vi "Assist Sampling Setup Panel.vi"(8 "error in":errorcluster, 10 "fs in [Hz]":dbl, 11 "session in":T2={"adc"={"niScope"={"channel cfg"=[], "sessions"=[], "multi cards"=FALSE, "channels"=0, "type"=enum."n/a", "memory [B/chn]"=0, "ext. clock [Hz]"=0.0, "samples count"=0, "use streaming"=FALSE, "proc setup"={"packet size [smpl]"=0, "current timeout [s]"=0.0, "blk2blk timeout [s]"=0.0, "event time"=timestamp(0 s since 1904-01-01), "temp sampl T [s]"=0.0, "data queue"=refnum, "stop notifier"=refnum, "proc ref"=refnum}, "sample width [B]"=0, "ranges [V]"=[], "trigger setup"={"coupling"=1, "level [V]"=0.0, "slope"=0, "mode"=enum."Immediate"}, "fs [Hz]"=0.0, "bitres [bit]"=0}, "3458A"={"channels"=[], "sync unit"={"VISA"="", "type"=enum."Picotest U6200A"}, "awg unit"={"type"=enum."Agilent 331xxA to 332xxA", "VISA"="", "enable 10MHz ref"=FALSE}, "sync mode"=enum."MASTER-SLAVE, MASTER clocked by TIMER", "streaming mode"=FALSE, "idn mode"=enum."Auto", "sampling mode"=enum."DCV", "Ts [s]"=0.0, "sample memory [B]"=0, "proc setup"={"channel id"=0, "packet size [smpl]"=0, "current timeout [s]"=0.0, "blk2blk timeout [s]"=0.0, "event time"=timestamp(0 s since 1904-01-01), "stop notifier"=refnum, "data queues"=[], "proc refs"=[], "bus semaphore"=refnum}, "sample size [B]"=0, "sample count"=0, "aux data"={"channel id"=0, "valid?"=[], "gain [V]"=[], "timestamp [s]"=[], "Ts [s]"=0.0, "abs timestamp"=timestamp(0 s since 1904-01-01), "t [deg C]"=[]}, "ranges [V]"=[], "aperture [s]"=0.0, "LEVEL trigger"={"edge"=enum."POS", "level [V]"=0.0, "coupling"=enum."DC"}, "trigger mode"=enum."AUTO", "measure temp.?"=FALSE, "disp mesages"=[], "shared bus?"=FALSE, "disable display?"=FALSE, "aper mode"=enum."Manual", "aper rules"=[]}, "dsdll"={"dsdll"={"dsdll path"=path "", "dsdll handle"=[], "output devices"=[], "capture devices"=[]}, "channels"=0, "device id"=0, "channel idns"=[], "proc setup"={"packet size [smpl]"=0, "current timeout [s]"=0.0, "blk2blk timeout [s]"=0.0, "event time"=timestamp(0 s since 1904-01-01), "data queue"=refnum, "stop notifier"=refnum, "proc ref"=refnum}, "samples count"=0, "fs [Hz]"=0.0}, "type"=enum."niScope", "channel idn str"=[], "aux instr idn str"=[], "modified?"=FALSE, "simadc"={"channels"=[], "range [V]"=0.0, "Ts step [s]"=0.0, "time [s]"=0.0, "fs [Hz]"=0.0, "count"=0, "smpl offset"=0, "set count"=0, "bit res"=0}, "force rst?"=FALSE, "exit mode"=enum."Immediate reset", "exit dly"=0.0, "exit tmr"=timestamp(0 s since 1904-01-01), "busy?"=FALSE, "accessed?"=FALSE, "QuADC session"={"channel cfg"=[], "sessions"=[], "multi cards"=FALSE, "channels"=0, "type"=enum."n/a", "memory [B/chn]"=0, "ext. clock [Hz]"=0.0, "samples count"=0, "use streaming"=FALSE, "proc setup"={"packet size [smpl]"=0, "current timeout [s]"=0.0, "blk2blk timeout [s]"=0.0, "event time"=timestamp(0 s since 1904-01-01), "temp sampl T [s]"=0.0, "data queue"=refnum, "stop notifier"=refnum, "proc ref"=refnum}, "sample width [B]"=0, "ranges [V]"=[], "trigger setup"={"coupling"=1, "level [V]"=0.0, "slope"=0, "mode"=enum."Immediate"}, "fs [Hz]"=0.0, "bitres [bit]"=0}}, "sequence"=[], "sequence setup"={"group setups"=[], "average cycles"=0, "range mode"=enum."Keep defaults", "fs mode"=enum."Frequency", "rng even"=0.0, "rng odd"=0.0, "folder"=path "", "name base"="", "meas id"=0, "settle [s]"=0.0}, "golpi"=refnum, "processing setup"={"mode"=enum."Raw", "call after avgs?"=FALSE, "calculate?"=FALSE, "raw mode"={"command"="", "result mode"=enum."Display console output (only Octave)", "res variable"=""}, "QWTB"={"QWTB path"=path "", "alg filter path"="", "alg ids"=[], "alg parameters"=[], "parsed parameters"=[], "selected alg id"="", "selected unc mode"=enum."None", "qwtb mcc"=100, "qwtb timeout"=90, "qwtb covg"=95.0, "qwtb ofs"=0, "qwtb lim data"=0, "multicore"={"jobs folder"=path "", "cores"=0, "max jobs"=0, "mode"=enum."Singlecore"}, "unc once?"=FALSE}}, "corrections"={"transducers"={"channels"=[], "last path"=path ""}, "digitizer"={"last path"=path "", "channel paths"=[], "channel idns"=[], "correction name"="", "channel names"=[], "folders to copy"=[], "channel valid"=[], "correction path"=path "", "correction rel path"="", "rel folders to copy"=[]}}, "assist cfg"={"P"=0, "Q"=0, "rel shift"=0.0, "ref freq"=0.0, "min fs"=0.0, "max fs tol"=0.0, "min int"=0.0, "max int"=0.0, "max err"=0.0, "max timeout"=0.0}} {"corrections"."transducers"."channels"."Phase index" min=1 step=1; "adc"."QuADC session"."trigger setup"."level [V]" format="%.2f"; "adc"."QuADC session"."trigger setup"."coupling" items=["AC"=0, "DC"=1, "HF Reject"=3, "LF Reject"=4, "AC Plus HF Reject"=1001]; "adc"."QuADC session"."channel cfg"."Clock fr. (Hz)" min=0.0 format="%#_9p"; "adc"."QuADC session"."channel cfg"."Number of JJ" min=1; "adc"."QuADC session"."channel cfg"."Range [Vpk]" min=0.0; "adc"."QuADC session"."channel cfg"."Channel" min=0; "adc"."3458A"."channels"."Range [Vpk]" min=0.0; "adc"."niScope"."trigger setup"."level [V]" format="%.2f"; "adc"."niScope"."trigger setup"."coupling" items=["AC"=0, "DC"=1, "HF Reject"=3, "LF Reject"=4, "AC Plus HF Reject"=1001]; "adc"."niScope"."channel cfg"."Range [Vpk]" min=0.0; "adc"."niScope"."channel cfg"."Channel" min=0}) -> (0 "error out":errorcluster, 1 "ok":bool, 2 "smpl setup":T1, 3 "session out":T2={"adc"={"niScope"={"channel cfg"=[], "sessions"=[], "multi cards"=FALSE, "channels"=0, "type"=enum."n/a", "memory [B/chn]"=0, "ext. clock [Hz]"=0.0, "samples count"=0, "use streaming"=FALSE, "proc setup"={"packet size [smpl]"=0, "current timeout [s]"=0.0, "blk2blk timeout [s]"=0.0, "event time"=timestamp(0 s since 1904-01-01), "temp sampl T [s]"=0.0, "data queue"=refnum, "stop notifier"=refnum, "proc ref"=refnum}, "sample width [B]"=0, "ranges [V]"=[], "trigger setup"={"coupling"=1, "level [V]"=0.0, "slope"=0, "mode"=enum."Immediate"}, "fs [Hz]"=0.0, "bitres [bit]"=0}, "3458A"={"channels"=[], "sync unit"={"VISA"="", "type"=enum."Picotest U6200A"}, "awg unit"={"type"=enum."Agilent 331xxA to 332xxA", "VISA"="", "enable 10MHz ref"=FALSE}, "sync mode"=enum."MASTER-SLAVE, MASTER clocked by TIMER", "streaming mode"=FALSE, "idn mode"=enum."Auto", "sampling mode"=enum."DCV", "Ts [s]"=0.0, "sample memory [B]"=0, "proc setup"={"channel id"=0, "packet size [smpl]"=0, "current timeout [s]"=0.0, "blk2blk timeout [s]"=0.0, "event time"=timestamp(0 s since 1904-01-01), "stop notifier"=refnum, "data queues"=[], "proc refs"=[], "bus semaphore"=refnum}, "sample size [B]"=0, "sample count"=0, "aux data"={"channel id"=0, "valid?"=[], "gain [V]"=[], "timestamp [s]"=[], "Ts [s]"=0.0, "abs timestamp"=timestamp(0 s since 1904-01-01), "t [deg C]"=[]}, "ranges [V]"=[], "aperture [s]"=0.0, "LEVEL trigger"={"edge"=enum."POS", "level [V]"=0.0, "coupling"=enum."DC"}, "trigger mode"=enum."AUTO", "measure temp.?"=FALSE, "disp mesages"=[], "shared bus?"=FALSE, "disable display?"=FALSE, "aper mode"=enum."Manual", "aper rules"=[]}, "dsdll"={"dsdll"={"dsdll path"=path "", "dsdll handle"=[], "output devices"=[], "capture devices"=[]}, "channels"=0, "device id"=0, "channel idns"=[], "proc setup"={"packet size [smpl]"=0, "current timeout [s]"=0.0, "blk2blk timeout [s]"=0.0, "event time"=timestamp(0 s since 1904-01-01), "data queue"=refnum, "stop notifier"=refnum, "proc ref"=refnum}, "samples count"=0, "fs [Hz]"=0.0}, "type"=enum."niScope", "channel idn str"=[], "aux instr idn str"=[], "modified?"=FALSE, "simadc"={"channels"=[], "range [V]"=0.0, "Ts step [s]"=0.0, "time [s]"=0.0, "fs [Hz]"=0.0, "count"=0, "smpl offset"=0, "set count"=0, "bit res"=0}, "force rst?"=FALSE, "exit mode"=enum."Immediate reset", "exit dly"=0.0, "exit tmr"=timestamp(0 s since 1904-01-01), "busy?"=FALSE, "accessed?"=FALSE, "QuADC session"={"channel cfg"=[], "sessions"=[], "multi cards"=FALSE, "channels"=0, "type"=enum."n/a", "memory [B/chn]"=0, "ext. clock [Hz]"=0.0, "samples count"=0, "use streaming"=FALSE, "proc setup"={"packet size [smpl]"=0, "current timeout [s]"=0.0, "blk2blk timeout [s]"=0.0, "event time"=timestamp(0 s since 1904-01-01), "temp sampl T [s]"=0.0, "data queue"=refnum, "stop notifier"=refnum, "proc ref"=refnum}, "sample width [B]"=0, "ranges [V]"=[], "trigger setup"={"coupling"=1, "level [V]"=0.0, "slope"=0, "mode"=enum."Immediate"}, "fs [Hz]"=0.0, "bitres [bit]"=0}}, "sequence"=[], "sequence setup"={"group setups"=[], "average cycles"=0, "range mode"=enum."Keep defaults", "fs mode"=enum."Frequency", "rng even"=0.0, "rng odd"=0.0, "folder"=path "", "name base"="", "meas id"=0, "settle [s]"=0.0}, "golpi"=refnum, "processing setup"={"mode"=enum."Raw", "call after avgs?"=FALSE, "calculate?"=FALSE, "raw mode"={"command"="", "result mode"=enum."Display console output (only Octave)", "res variable"=""}, "QWTB"={"QWTB path"=path "", "alg filter path"="", "alg ids"=[], "alg parameters"=[], "parsed parameters"=[], "selected alg id"="", "selected unc mode"=enum."None", "qwtb mcc"=100, "qwtb timeout"=90, "qwtb covg"=95.0, "qwtb ofs"=0, "qwtb lim data"=0, "multicore"={"jobs folder"=path "", "cores"=0, "max jobs"=0, "mode"=enum."Singlecore"}, "unc once?"=FALSE}}, "corrections"={"transducers"={"channels"=[], "last path"=path ""}, "digitizer"={"last path"=path "", "channel paths"=[], "channel idns"=[], "correction name"="", "channel names"=[], "folders to copy"=[], "channel valid"=[], "correction path"=path "", "correction rel path"="", "rel folders to copy"=[]}}, "assist cfg"={"P"=0, "Q"=0, "rel shift"=0.0, "ref freq"=0.0, "min fs"=0.0, "max fs tol"=0.0, "min int"=0.0, "max int"=0.0, "max err"=0.0, "max timeout"=0.0}} {"corrections"."transducers"."channels"."Phase index" min=1 step=1; "adc"."QuADC session"."trigger setup"."level [V]" format="%.2f"; "adc"."QuADC session"."trigger setup"."coupling" items=["AC"=0, "DC"=1, "HF Reject"=3, "LF Reject"=4, "AC Plus HF Reject"=1001]; "adc"."QuADC session"."channel cfg"."Clock fr. (Hz)" min=0.0 format="%#_9p"; "adc"."QuADC session"."channel cfg"."Number of JJ" min=1; "adc"."QuADC session"."channel cfg"."Range [Vpk]" min=0.0; "adc"."QuADC session"."channel cfg"."Channel" min=0; "adc"."3458A"."channels"."Range [Vpk]" min=0.0; "adc"."niScope"."trigger setup"."level [V]" format="%.2f"; "adc"."niScope"."trigger setup"."coupling" items=["AC"=0, "DC"=1, "HF Reject"=3, "LF Reject"=4, "AC Plus HF Reject"=1001]; "adc"."niScope"."channel cfg"."Range [Vpk]" min=0.0; "adc"."niScope"."channel cfg"."Channel" min=0})   [LabVIEW 2018]
uses:
  Meas Session.ctl
  adc/ADC Session.ctl
  drivers/niScope/niScope Session.ctl
  drivers/niScope/niScope Virtual Channel Config.ctl
  drivers/niScope/niScope Virtual Channel Mode.ctl
  drivers/niScope/niScope Virtual Channel Input Z.ctl
  drivers/niScope/niScope Virtual Channel Coupling.ctl
  drivers/niScope/niScope Type.ctl
  drivers/niScope/niScope Digitizing Process Options.ctl
  drivers/niScope/niScope Data Packet.ctl
  drivers/niScope/niScope Trigger Setup.ctl
  <instrlib>/niScope/Controls/niScope trigger coupling.ctl
  <instrlib>/niScope/Controls/niScope trigger slope.ctl
  drivers/DMM/3458A Digitizer Session.ctl
  drivers/DMM/3458A Virtual Channel Config.ctl
  drivers/Counter/Counter Session.ctl
  drivers/Counter/Counter Type.ctl
  drivers/AWG/AWG Session.ctl
  drivers/AWG/AWG Type.ctl
  drivers/DMM/3458A Sync Mode.ctl
  drivers/DMM/3458A Idn Mode.ctl
  drivers/DMM/3458A Digitizing Low Levels/Configure/Sampling Mode.ctl
  drivers/DMM/3458A Digitizing Process Options.ctl
  drivers/DMM/3458A Data Packet.ctl
  drivers/DMM/3458A Aux Record Data.ctl
  drivers/DMM/3458A Digitizing Low Levels/Configure/Level Setup.ctl
  drivers/DMM/3458A Digitizing Low Levels/Configure/First Sample Trigger.ctl
  drivers/DMM/3458A Aperture Selection Mode.ctl
  drivers/dsdll/DSDLL Session.ctl
  drivers/dsdll/dsdll source distribution/dsdll_instance.ctl
  drivers/dsdll/dsdll source distribution/dsdll_device_record.ctl
  drivers/dsdll/DSDLL Process Config.ctl
  drivers/dsdll/DSDLL Data Packet.ctl
  adc/ADC Type.ctl
  drivers/simulated_adc/SimAdc Config.ctl
  drivers/simulated_adc/SimAdc Channel Cfg.ctl
  adc/ADC On Close Action.ctl
  drivers/Quatsch_driver/QuADCDriver/QuADC Session.ctl
  drivers/Quatsch_driver/QuADCDriver/QuADC Virtual Channel Config.ctl
  drivers/Quatsch_driver/QuADCDriver/QuADC Virtual Channel Mode.ctl
  drivers/Quatsch_driver/QuADCDriver/QuADC Virtual Channel Input Z.ctl
  drivers/Quatsch_driver/QuADCDriver/QuADC Virtual Channel Coupling.ctl
  drivers/Quatsch_driver/QuADCDriver/QuADC Type.ctl
  drivers/Quatsch_driver/QuADCDriver/QuADC Digitizing Process Options.ctl
  drivers/Quatsch_driver/QuADCDriver/QuADC Data Packet.ctl
  drivers/Quatsch_driver/QuADCDriver/QuADC Trigger Setup.ctl
  Meas Sequence Item.ctl
  Meas Sampling Configuration.ctl
  adc/ADC Trig Config.ctl
  adc/ADC Trig Mode Source.ctl
  adc/ADC Trig Coupling.ctl
  adc/ADC Trig Slope.ctl
  processing/QWTB/Meas Proc QWTB Algorithm Parameter Data.ctl
  Meas Sequence Configuration.ctl
  Meas Range Mode.ctl
  Meas Sampling Rate Mode.ctl
  octave/golpi/mpc/golpi_session_ref.ctl
  octave/golpi/mpc/golpi_session.ctl
  octave/golpi/GOLPI Library.lvlibp/Public/GOLPI reference Type Def.ctl
  octave/golpi/GOLPI Library.lvlibp/LV Process source distribution/Pipe Handle.ctl
  processing/Meas Process Config.ctl
  processing/Meas Process Mode.ctl
  processing/Meas Process Raw Config.ctl
  processing/Meas Process Raw Result Mode.ctl
  processing/QWTB/Meas Proc QWTB Setup.ctl
  processing/QWTB/Meas Proc QWTB Uncertainty Mode.ctl
  processing/QWTB/Meas Proc QWTB Multicore Setup.ctl
  processing/QWTB/Meas Proc QWTB Multicore Type.ctl
  Corrections/Corr Setup.ctl
  Corrections/Corr Tranducer Item.ctl
  Corrections/Corr Digitizers.ctl
  Assist Panel Setup.ctl
  Assist Sampling Setup.ctl
  Assist Coherent Sampling Finder Setup.ctl
  adc/ADC Sampling Rate Step Mode.ctl
  varilib/varilib.lvlib
  drivers/niScope/niScope Virtual Digitizer.lvlib
  drivers/DMM/3458A Virtual Digitizer.lvlib
  drivers/Counter/Counter.lvlib
  drivers/AWG/AWG.lvlib
  drivers/DMM/3458A Digitizing Low Levels/3458A Digitizing Low Levels.lvlib
  drivers/dsdll/DSDLL Virtual Digitizer.lvlib
  octave/golpi/GOLPI Library.lvlibp/LV Process source distribution/LV Process library.lvlib
  octave/golpi/GOLPI Library.lvlibp
  octave/golpi/mpc/GOLPI Multi Process.lvlib
  drivers/Quatsch_driver/QuADCDriver/QuADC Virtual Digitizer.lvlib
  drivers/dsdll/dsdll source distribution/dsdll.lvlib
panel:
  out "found harm dist":dbl=10000.0 caption="Harmonics dist.  [bin]" format="%#_4p"
  out "found bin step":dbl=10000.0 caption="DFT bin step [Hz]" format="%#_4p"
  in  "rel shift":dbl caption="Relative shift [ppm]"
  out "found error":dbl=10000.0 caption="Relative error [-]" format="%#_3g"
  out "per mode":bool
  in  "btn cancel":bool
  in  "btn ok":bool
  out "found periods":dbl=10000.0 caption="Periods count [-]" format="%#_4p"
  out "found int":dbl=10000.0 caption="Integration time [s]" format="%#_4p"
  out "smpl count":i64=10000 caption="Samples count"
  out "found fs":dbl=10000.0 caption="Found fs [Hz]" format="%#_8p"
  in  "btn rough":bool
  in  "btn coh":bool
  in  "max periods":dbl=20.0 caption="Max periods [-]" format="%#_8p"
  in  "min periods":dbl=10.0 caption="Min periods [-]" format="%#_8p"
  in  "max timeout":dbl=5.0 caption="Max timeout [s]" format="%#_8g"
  in  "max err":dbl=1e-09 caption="Max setup error [-]" format="%#_8g"
  in  "max int":dbl=0.2 caption="Max integration t. [s]" format="%#_4p"
  in  "min int":dbl=10000.0 caption="Min integration t. [s]" format="%#_4p"
  out "max adc fs":dbl=10000.0 caption="Max ADC fs [Hz]" format="%#_8p"
  out "min adc fs":dbl=10000.0 caption="Min ADC fs [Hz]" format="%#_8p"
  out "max fs":dbl caption="Maximum fs [Hz]" format="%#_6p"
  in  "max fs rel tol":dbl=0.5 caption="fs max tolerance [-]"
  in  "min fs":dbl=10000.0 caption="Minimum fs [Hz]" format="%#_8p"
  out "f0":dbl caption="Fundamental frequency f0 [Hz]" format="%#_9p"
  in  "Q":i32
  in  "P":i32
  in  "btn meas":bool
  in  "ref freq":dbl caption="Reference frequency fr [Hz]" format="%#_9p"
  # "f0 = fr*P/Q*\n*(1 + shift)"
  # "ADC:"
  # "IP Address"
  # "."
  # "."
  # "."
  # ":"
  # "ADC:"
  # "IP Address"
  # "."
  # "."
  # "."
  # ":"
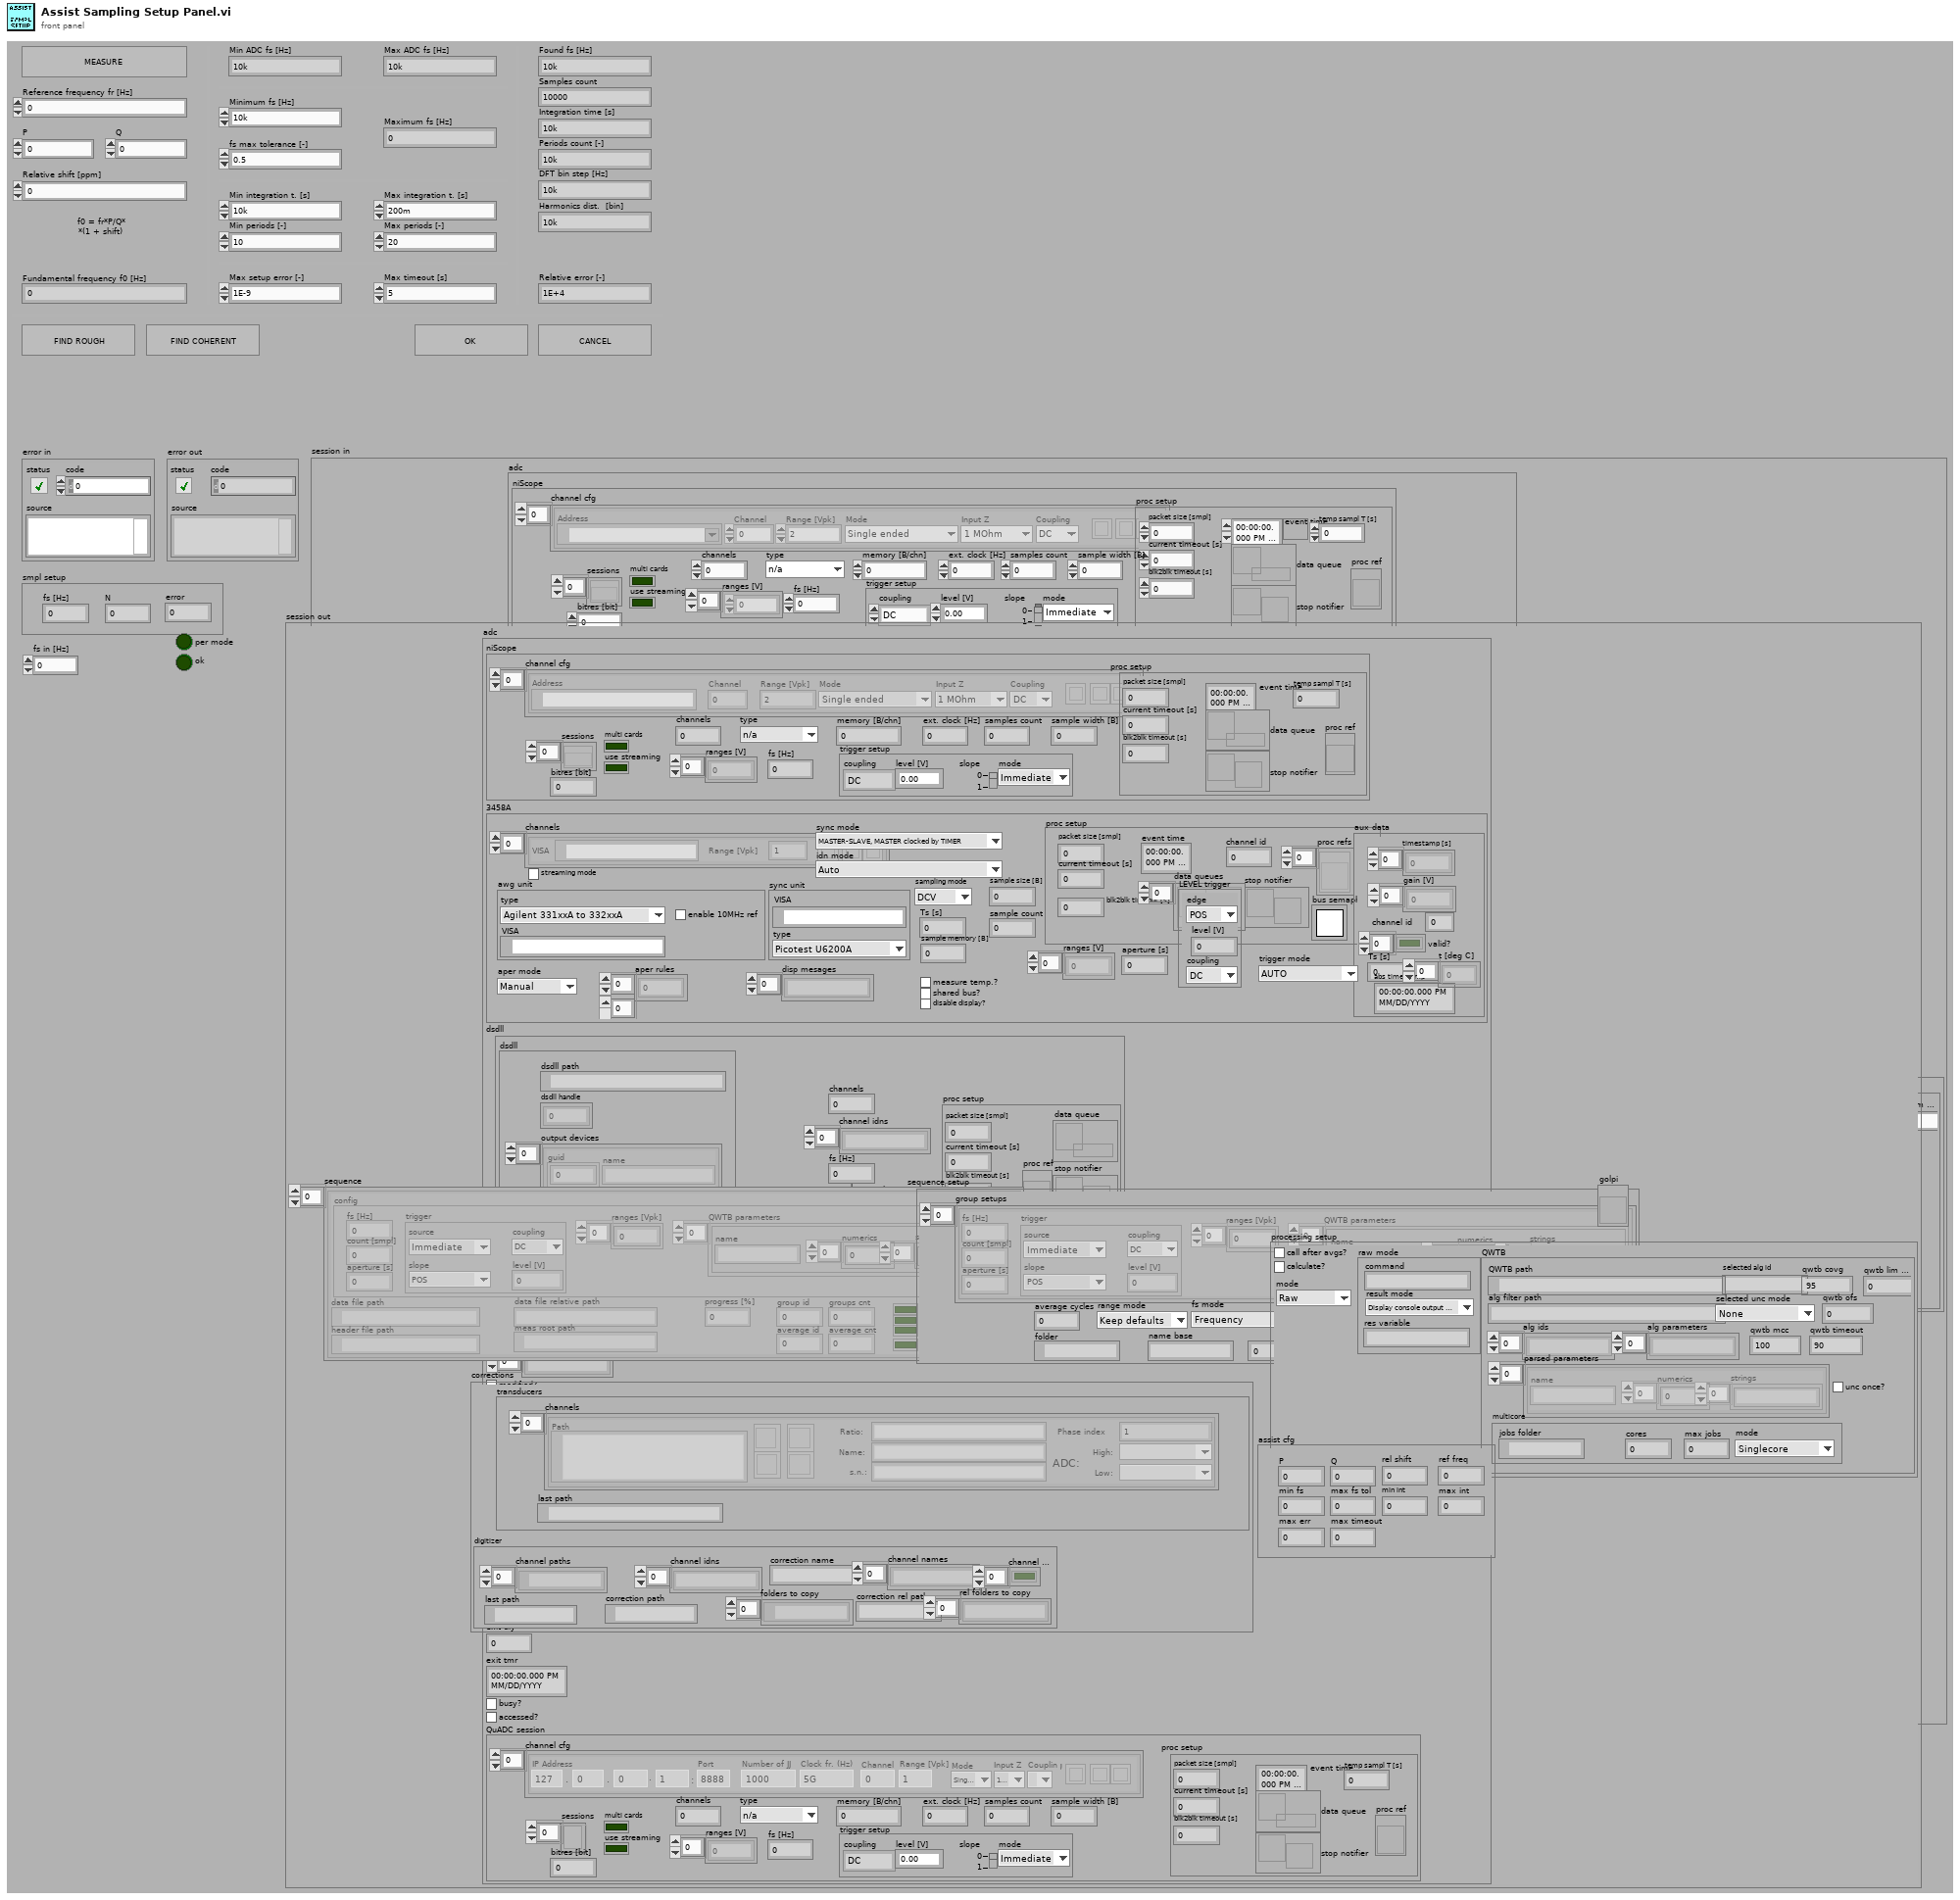
[diagram p1: front panel]
types:
  T1 = typedef "Assist Sampling Setup.ctl" = cluster{"fs [Hz]":ext, "N":i64, "error":dbl}
  T2 = typedef "Meas Session.ctl" = cluster{"adc":T3, "sequence":T45[], "sequence setup":T52, "golpi":T55, "processing setup":T56, "corrections":T64, "assist cfg":T67}
  T3 = typedef "ADC Session.ctl" = cluster{"niScope":T4, "3458A":T14, "dsdll":T29, "type":T33, "channel idn str":string[], "aux instr idn str":string[], "modified?":bool, "simadc":T34, "force rst?":bool, "exit mode":T36, "exit dly":dbl, "exit tmr":timestamp, "busy?":bool, "accessed?":bool, "QuADC session":T37}
  T4 = typedef "niScope Virtual Digitizer.lvlib/niScope Session.ctl" = cluster{"channel cfg":T5[], "sessions":refnum<k20>[], "multi cards":bool, "channels":i32, "type":T9, "memory [B/chn]":i32, "ext. clock [Hz]":dbl, "samples count":i64, "use streaming":bool, "proc setup":T10, "sample width [B]":i32, "ranges [V]":dbl[], "trigger setup":T11, "fs [Hz]":dbl, "bitres [bit]":i32}
  T5 = typedef "niScope Virtual Digitizer.lvlib/niScope Virtual Channel Config.ctl" = cluster{"Address":refnum<k15>, "Channel":i32, "Mode":T6, "Input Z":T7, "Coupling":T8, "Range [Vpk]":dbl, "btn clr":bool, "btn up":bool, "btn down":bool}
  T6 = typedef "niScope Virtual Digitizer.lvlib/niScope Virtual Channel Mode.ctl" = enum16{"Single ended", "Unbal. differential", "Differential"}
  T7 = typedef "niScope Virtual Digitizer.lvlib/niScope Virtual Channel Input Z.ctl" = enum16{"1 MOhm", "50 Ohm"}
  T8 = typedef "niScope Virtual Digitizer.lvlib/niScope Virtual Channel Coupling.ctl" = enum16{"AC", "DC", "GND"}
  T9 = typedef "niScope Virtual Digitizer.lvlib/niScope Type.ctl" = enum16{"n/a", "5922"}
  T10 = typedef "niScope Virtual Digitizer.lvlib/niScope Digitizing Process Options.ctl" = cluster{"packet size [smpl]":i64, "current timeout [s]":dbl, "blk2blk timeout [s]":dbl, "event time":timestamp, "temp sampl T [s]":dbl, "data queue":refnum<queue>, "stop notifier":refnum<notifier>, "proc ref":refnum<vi>}
  T11 = typedef "niScope Virtual Digitizer.lvlib/niScope Trigger Setup.ctl" = cluster{"coupling":T12, "level [V]":dbl, "slope":T13, "mode":enum16{"Immediate", "External", "Level"}}
  T12 = typedef "niScope trigger coupling.ctl" = u16
  T13 = typedef "niScope trigger slope.ctl" = i32
  T14 = typedef "3458A Virtual Digitizer.lvlib/3458A Digitizer Session.ctl" = cluster{"channels":T15[], "sync unit":T16, "awg unit":T18, "sync mode":T20, "streaming mode":bool, "idn mode":T21, "sampling mode":T22, "Ts [s]":dbl, "sample memory [B]":i32, "proc setup":T23, "sample size [B]":i32, "sample count":i32, "aux data":T25, "ranges [V]":dbl[], "aperture [s]":dbl, "LEVEL trigger":T26, "trigger mode":T27, "measure temp.?":bool, "disp mesages":string[], "shared bus?":bool, "disable display?":bool, "aper mode":T28, "aper rules":dbl[][]}
  T15 = typedef "3458A Virtual Digitizer.lvlib/3458A Virtual Channel Config.ctl" = cluster{"VISA":refnum<visa-resource-name>, "Range [Vpk]":dbl, "btn clr":bool, "btn up":bool, "btn down":bool}
  T16 = typedef "Counter.lvlib/Counter Session.ctl" = cluster{"VISA":refnum<visa-resource-name>, "type":T17}
  T17 = typedef "Counter.lvlib/Counter Type.ctl" = enum16{"Picotest U6200A", "dummy"}
  T18 = typedef "AWG.lvlib/AWG Session.ctl" = cluster{"type":T19, "VISA":refnum<visa-resource-name>, "enable 10MHz ref":bool}
  T19 = typedef "AWG.lvlib/AWG Type.ctl" = enum16{"Agilent 331xxA to 332xxA", "Agilent 335xxA to 336xxA", "Tektronix AFG3101C", "dummy"}
  T20 = typedef "3458A Virtual Digitizer.lvlib/3458A Sync Mode.ctl" = enum16{"MASTER-SLAVE, MASTER clocked by TIMER", "MASTER-SLAVE, MASTER clocked by AWG", "ALL clocked by AWG", "MASTER-SLAVE, ALL clocked by TIMER", "ALL clocked by AWG with DFLL"}
  T21 = typedef "3458A Virtual Digitizer.lvlib/3458A Idn Mode.ctl" = enum16{"Auto", "Sequential (chn A, chn B, ...)", "From calibration string"}
  T22 = typedef "3458A Virtual Digitizer.lvlib/3458A Digitizing Low Levels.lvlib/Sampling Mode.ctl" = enum16{"DCV", "DSDC", "DSAC"}
  T23 = typedef "3458A Virtual Digitizer.lvlib/3458A Digitizing Process Options.ctl" = cluster{"channel id":i32, "packet size [smpl]":i32, "current timeout [s]":dbl, "blk2blk timeout [s]":dbl, "event time":timestamp, "stop notifier":refnum<notifier>, "data queues":refnum<queue>[], "proc refs":refnum<vi>[], "bus semaphore":T24}
  T24 = typedef "Semaphore RefNum" = refnum<k1>
  T25 = typedef "3458A Virtual Digitizer.lvlib/3458A Aux Record Data.ctl" = cluster{"channel id":i32, "valid?":bool[], "gain [V]":dbl[], "timestamp [s]":dbl[], "Ts [s]":dbl, "abs timestamp":timestamp, "t [deg C]":dbl[]}
  T26 = typedef "3458A Virtual Digitizer.lvlib/3458A Digitizing Low Levels.lvlib/Level Setup.ctl" = cluster{"edge":enum16{"POS", "NEG"}, "level [V]":dbl, "coupling":enum16{"DC", "AC"}}
  T27 = typedef "3458A Virtual Digitizer.lvlib/3458A Digitizing Low Levels.lvlib/First Sample Trigger.ctl" = enum16{"AUTO", "EXT", "SYN", "SGL", "HOLD", "LEVEL"}
  T28 = typedef "3458A Virtual Digitizer.lvlib/3458A Aperture Selection Mode.ctl" = enum16{"Manual", "Maximum", "Table"}
  T29 = typedef "DSDLL Virtual Digitizer.lvlib/DSDLL Session.ctl" = cluster{"dsdll":T30, "channels":i32, "device id":i32, "channel idns":string[], "proc setup":T32, "samples count":i32, "fs [Hz]":dbl}
  T30 = typedef "dsdll.lvlib/dsdll_instance.ctl" = cluster{"dsdll path":path, "dsdll handle":u8[], "output devices":T31[], "capture devices":T31[]}
  T31 = typedef "dsdll.lvlib/dsdll_device_record.ctl" = cluster{"guid":u8[], "name":string}
  T32 = typedef "DSDLL Virtual Digitizer.lvlib/DSDLL Process Config.ctl" = cluster{"packet size [smpl]":i32, "current timeout [s]":dbl, "blk2blk timeout [s]":dbl, "event time":timestamp, "data queue":refnum<queue>, "stop notifier":refnum<notifier>, "proc ref":refnum<vi>}
  T33 = typedef "ADC Type.ctl" = enum16{"niScope", "3458A", "DirectSound DLL", "dummy", "QuADC"}
  T34 = typedef "SimAdc Config.ctl" = cluster{"channels":T35[], "range [V]":dbl, "Ts step [s]":dbl, "time [s]":dbl, "fs [Hz]":dbl, "count":i64, "smpl offset":i64, "set count":i64, "bit res":i32}
  T35 = typedef "SimAdc Channel Cfg.ctl" = cluster{"harmonics":dbl[][], "btn clear":bool, "noise":dbl, "fundamental [Hz]":dbl}
  T36 = typedef "ADC On Close Action.ctl" = enum16{"Immediate reset", "Delayed reset"}
  T37 = typedef "QuADC Virtual Digitizer.lvlib/QuADC Session.ctl" = cluster{"channel cfg":T38[], "sessions":refnum<k5>[], "multi cards":bool, "channels":i32, "type":T42, "memory [B/chn]":i32, "ext. clock [Hz]":dbl, "samples count":i64, "use streaming":bool, "proc setup":T43, "sample width [B]":i32, "ranges [V]":dbl[], "trigger setup":T44, "fs [Hz]":dbl, "bitres [bit]":i32}
  T38 = typedef "QuADC Virtual Digitizer.lvlib/QuADC Virtual Channel Config.ctl" = cluster{"Channel":i32, "Mode":T39, "Input Z":T40, "Coupling":T41, "Range [Vpk]":dbl, "btn clr":bool, "btn up":bool, "btn down":bool, "IP address A":u8, "IP address B":u8, "IP address C":u8, "IP address D":u8, "Port":u16, "Number of JJ":u32, "Clock fr. (Hz)":dbl}
  T39 = typedef "QuADC Virtual Digitizer.lvlib/QuADC Virtual Channel Mode.ctl" = enum16{"Single ended", "Unbal. differential", "Differential"}
  T40 = typedef "QuADC Virtual Digitizer.lvlib/QuADC Virtual Channel Input Z.ctl" = enum16{"1 MOhm", "50 Ohm"}
  T41 = typedef "QuADC Virtual Digitizer.lvlib/QuADC Virtual Channel Coupling.ctl" = enum16{"AC", "DC", "GND"}
  T42 = typedef "QuADC Virtual Digitizer.lvlib/QuADC Type.ctl" = enum16{"n/a", "v1"}
  T43 = typedef "QuADC Virtual Digitizer.lvlib/QuADC Digitizing Process Options.ctl" = cluster{"packet size [smpl]":i64, "current timeout [s]":dbl, "blk2blk timeout [s]":dbl, "event time":timestamp, "temp sampl T [s]":dbl, "data queue":refnum<queue>, "stop notifier":refnum<notifier>, "proc ref":refnum<vi>}
  T44 = typedef "QuADC Virtual Digitizer.lvlib/QuADC Trigger Setup.ctl" = cluster{"coupling":T12, "level [V]":dbl, "slope":T13, "mode":enum16{"Immediate", "External", "Level"}}
  T45 = typedef "Meas Sequence Item.ctl" = cluster{"config":T46, "data file path":path, "header file path":path, "group id":i32, "average id":i32, "group done?":bool, "adc modified?":bool, "source modified?":bool, "progress [%]":dbl, "groups cnt":i32, "average cnt":i32, "data file relative path":string, "meas root path":path, "calculate?":bool}
  T46 = typedef "Meas Sampling Configuration.ctl" = cluster{"fs [Hz]":dbl, "count [smpl]":i64, "aperture [s]":dbl, "trigger":T47, "ranges [Vpk]":dbl[], "QWTB parameters":T51[]}
  T47 = typedef "ADC Trig Config.ctl" = cluster{"source":T48, "level [V]":dbl, "coupling":T49, "slope":T50}
  T48 = typedef "ADC Trig Mode Source.ctl" = enum16{"Immediate", "External", "Level"}
  T49 = typedef "ADC Trig Coupling.ctl" = enum16{"DC", "AC"}
  T50 = typedef "ADC Trig Slope.ctl" = enum16{"POS", "NEG"}
  T51 = typedef "Meas Proc QWTB Algorithm Parameter Data.ctl" = cluster{"name":string, "numerics":dbl[], "strings":string[]}
  T52 = typedef "Meas Sequence Configuration.ctl" = cluster{"group setups":T46[], "average cycles":i32, "range mode":T53, "fs mode":T54, "rng even":dbl, "rng odd":dbl, "folder":path, "name base":string, "meas id":i32, "settle [s]":dbl}
  T53 = typedef "Meas Range Mode.ctl" = enum16{"Keep defaults", "Set All channels", "Set Odd and Even channels"}
  T54 = typedef "Meas Sampling Rate Mode.ctl" = enum16{"Frequency", "Period"}
  T55 = typedef "GOLPI Multi Process.lvlib/golpi_session_ref.ctl" = refnum<vi>
  T56 = typedef "Meas Process Config.ctl" = cluster{"mode":T57, "call after avgs?":bool, "calculate?":bool, "raw mode":T58, "QWTB":T60}
  T57 = typedef "Meas Process Mode.ctl" = enum16{"Raw", "QWTB"}
  T58 = typedef "Meas Process Raw Config.ctl" = cluster{"command":string, "result mode":T59, "res variable":string}
  T59 = typedef "Meas Process Raw Result Mode.ctl" = enum16{"Display console output (only Octave)", "Display string variable", "Display result file %respath%"}
  T60 = typedef "Meas Proc QWTB Setup.ctl" = cluster{"QWTB path":path, "alg filter path":string, "alg ids":string[], "alg parameters":string[], "parsed parameters":T51[], "selected alg id":string, "selected unc mode":T61, "qwtb mcc":i32, "qwtb timeout":i32, "qwtb covg":dbl, "qwtb ofs":i64, "qwtb lim data":i64, "multicore":T62, "unc once?":bool}
  T61 = typedef "Meas Proc QWTB Uncertainty Mode.ctl" = enum16{"None", "GUF", "Monte Carlo"}
  T62 = typedef "Meas Proc QWTB Multicore Setup.ctl" = cluster{"jobs folder":path, "cores":i32, "max jobs":i32, "mode":T63}
  T63 = typedef "Meas Proc QWTB Multicore Type.ctl" = enum16{"Singlecore", "Multicore", "Multistation"}
  T64 = typedef "Corr Setup.ctl" = cluster{"transducers":cluster{"channels":T65[], "last path":path}, "digitizer":T66}
  T65 = typedef "Corr Tranducer Item.ctl" = cluster{"Path":path, "Ratio:":string, "Name:":string, "btn rem":bool, "btn up":bool, "btn down":bool, "s.n.:":string, "btn open":bool, "ratio o/i":dbl, "chn hi":u16, "chn lo":u16, "Phase index":i32}
  T66 = typedef "Corr Digitizers.ctl" = cluster{"last path":path, "channel paths":path[], "channel idns":string[], "correction name":string, "channel names":string[], "folders to copy":path[], "channel valid":bool[], "correction path":path, "correction rel path":string, "rel folders to copy":string[]}
  T67 = typedef "Assist Panel Setup.ctl" = cluster{"P":i32, "Q":i32, "rel shift":dbl, "ref freq":dbl, "min fs":dbl, "max fs tol":dbl, "min int":dbl, "max int":dbl, "max err":dbl, "max timeout":dbl}
  T68 = typedef "ADC Capabilities.ctl" = cluster{"max samples count":i64, "max fs [Hz]":ext, "min fs [Hz]":ext, "Ts step [s]":ext, "max Ts [s]":ext, "min Ts [s]":ext, "allows streaming?":bool, "streaming on?":bool, "has level trig?":bool, "has ext trig?":bool, "has aperture?":bool, "aper min [s]":dbl, "aper max [s]":dbl, "channels count":i32, "has ranges?":bool, "has temperature?":bool, "has temperature log?":bool, "has selfcal?":bool, "fs step [Hz]":ext, "smpl rate step mode":T69}
  T69 = typedef "ADC Sampling Rate Step Mode.ctl" = enum16{"const period", "const frequency"}
  T70 = typedef "Assist Coherent Sampling Finder Setup.ctl" = cluster{"fs min [Hz]":dbl, "fs rel tol [-]":dbl, "adc fs min [Hz]":dbl, "adc fs max [Hz]":dbl, "int min [s]":dbl, "int max [s]":dbl, "Ts step [s]":dbl, "fs step [Hz]":dbl, "timeout [s]":dbl, "max err [-]":dbl, "rate step mode":T69, "f0 [Hz]":dbl}
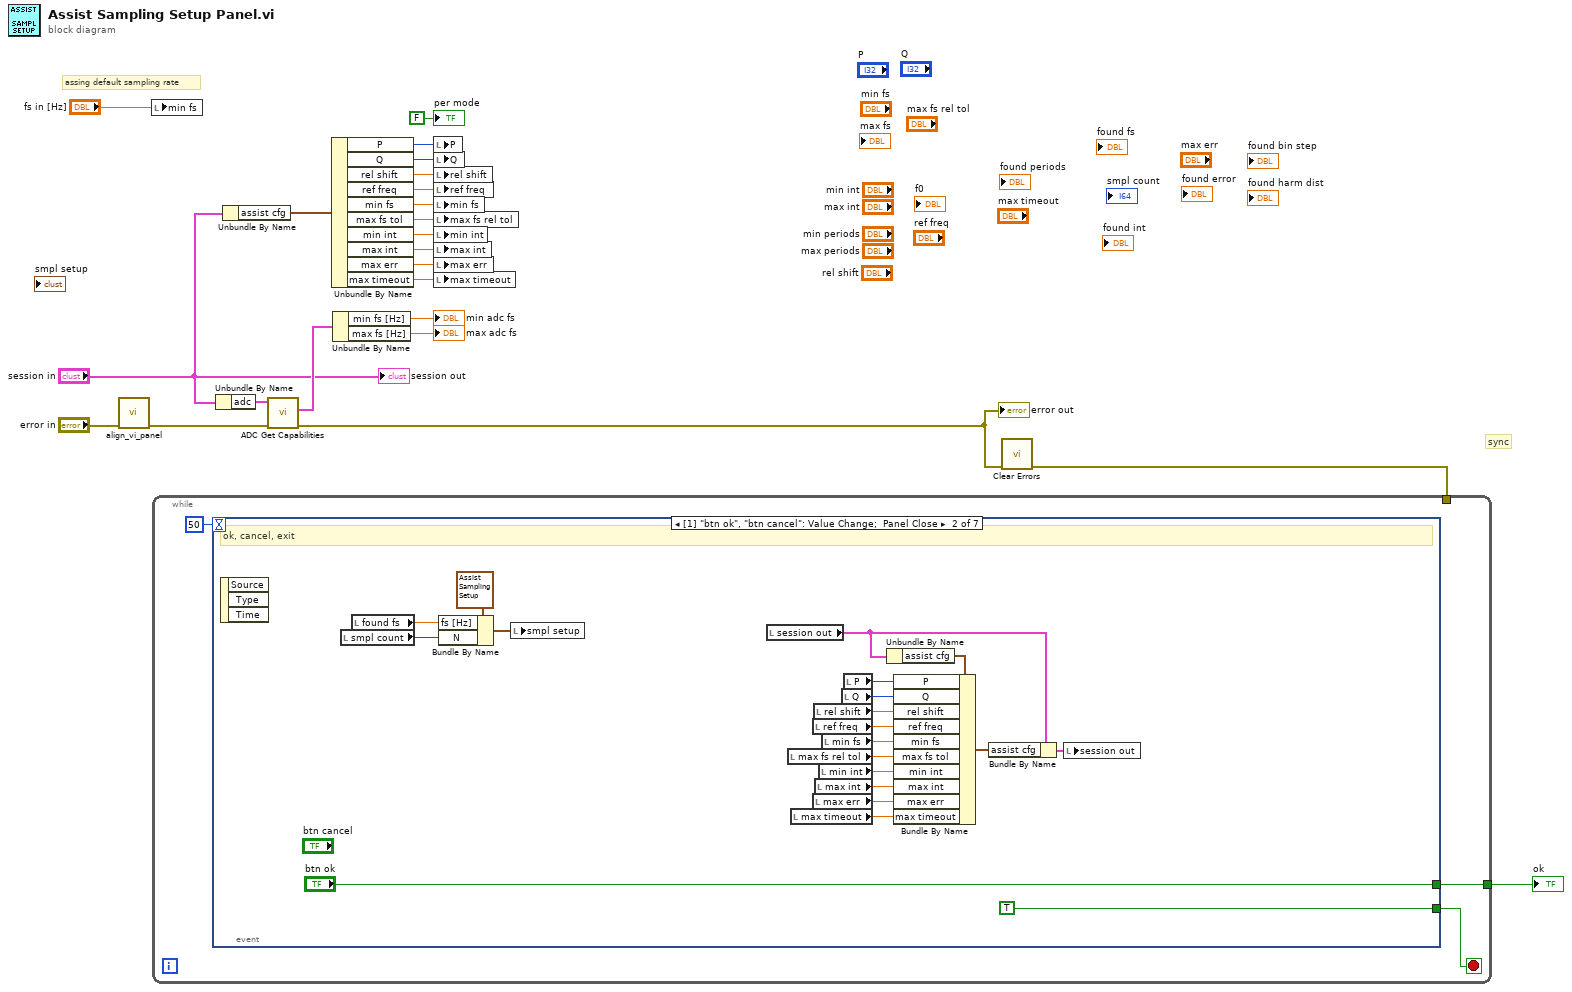
[diagram p0: block diagram]
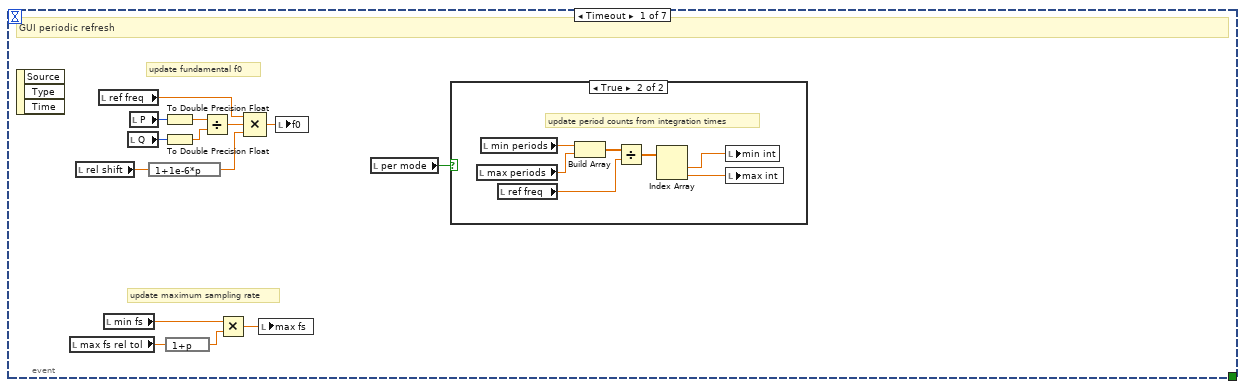
[diagram p2: hidden frame]
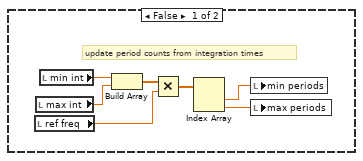
[diagram p3: hidden frame]
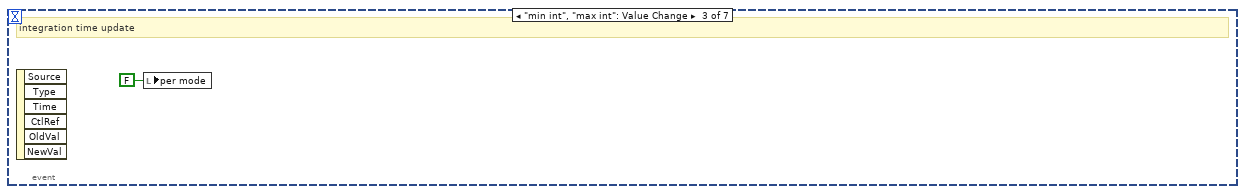
[diagram p4: hidden frame]
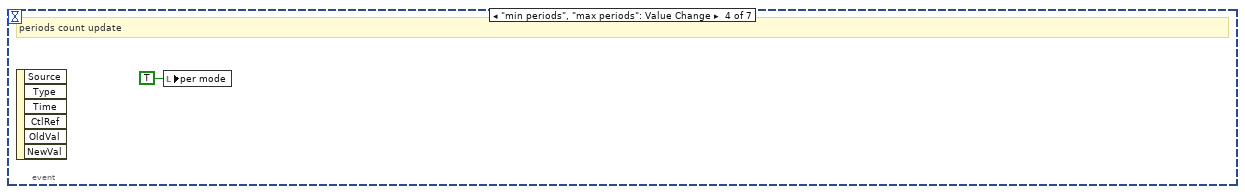
[diagram p5: hidden frame]
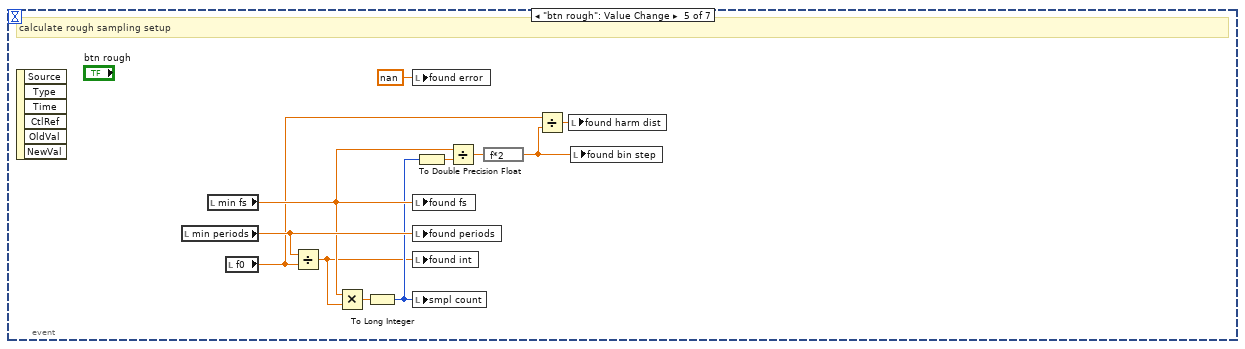
[diagram p6: hidden frame]
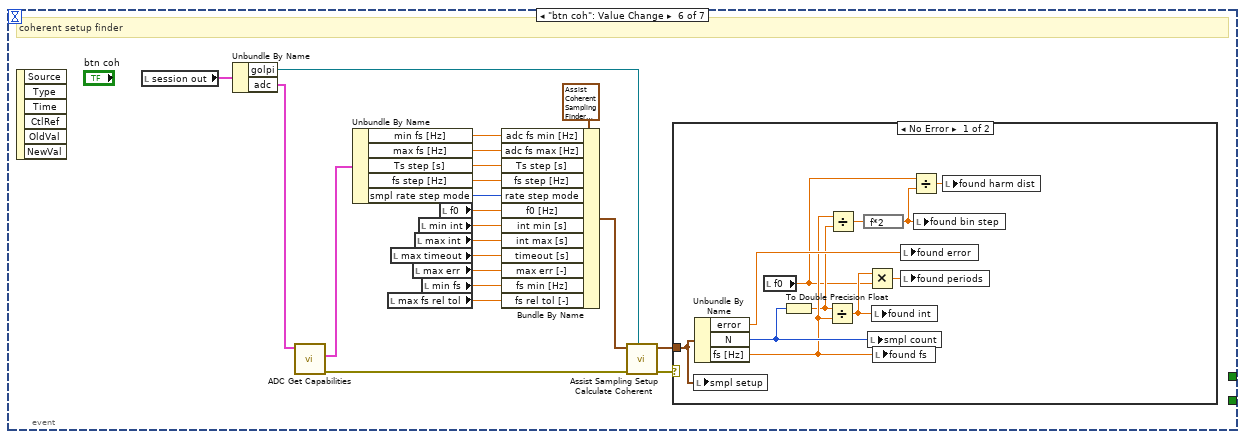
[diagram p7: hidden frame]
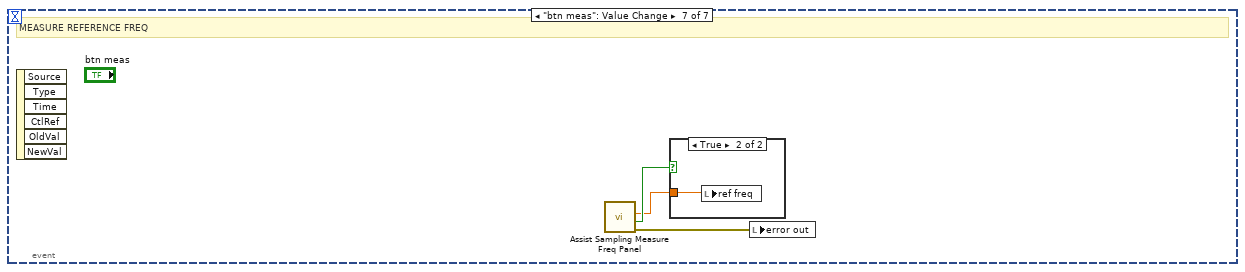
[diagram p9: hidden frame]
diagram:
  # "assing default sampling rate"
  # "sync"
  n1 = call "align_vi_panel.vi"("error in"="error in") -> ("error out"=w14:errorcluster)  [unwired: 10 in]
  n2 = local write "min fs"("fs in [Hz]") -> ()
  n3 = Unbundle By Name("session in") -> ("adc"=w23:T3)
  n4 = Unbundle By Name("session in") -> ("assist cfg"=w1:T67)
  n5 = call "ADC Get Capabilities.vi"("error in"=w14, "adc session in"=w23) -> ("error out"=w22:errorcluster, "capabilities"=w20:T68)  [unwired: 7 in, 1 out]
  "error out" <- w22
  n6 = Unbundle By Name(w1) -> ("P"=w13:i32, "Q"=w12:i32, "rel shift"=w11:dbl, "ref freq"=w10:dbl, "min fs"=w9:dbl, "max fs tol"=w8:dbl, "min int"=w7:dbl, "max int"=w6:dbl, "max err"=w5:dbl, "max timeout"=w4:dbl)
  n7 = Unbundle By Name(w20) -> ("min fs [Hz]"=→"min adc fs":ext, "max fs [Hz]"=→"max adc fs":ext)
  n8 = local write "P"(w13) -> ()
  n9 = local write "Q"(w12) -> ()
  n10 = local write "rel shift"(w11) -> ()
  n11 = local write "ref freq"(w10) -> ()
  n12 = local write "min fs"(w9) -> ()
  n13 = local write "max fs rel tol"(w8) -> ()
  n14 = local write "min int"(w7) -> ()
  n15 = local write "max int"(w6) -> ()
  n16 = local write "max err"(w5) -> ()
  n17 = local write "max timeout"(w4) -> ()
  n18 = call <vilib>:"Clear Errors.vi"("error in (no error)"=w22) -> ("error out"=w21:errorcluster)  [unwired: 5 in, 1 out]
  n19 = while {
    tunnel: w21 -> [_]
    tunnel: [w24] -> w17
    stop <- w25 stop-if-true
    n20 = event shown="[1] \"btn ok\", \"btn cancel\": Value Change;  Panel Close" {
      selector: _ -> [_ _ _ _ _ _ _]
      dyn-events: _ -> [_ _ _ _ _ _ _]
      timeout: 50 -> [_ _ _ _ _ _ _]
      tunnel: [_ TRUE _ _ _ _ _] -> w25
      tunnel: [_ "btn ok" _ _ _ _ _] -> w24
      event Timeout {
        # "update maximum sampling rate"
        # "update fundamental f0"
        # "GUI periodic refresh"
        n21 = event-data() -> ()  [unwired: 1 in, 3 out]
        n22 = local read "max fs rel tol"() -> (w33:dbl)
        n23 = local read "rel shift"() -> (w28:dbl)
        n24 = local read "ref freq"() -> (w35:dbl)
        n25 = local read "min fs"() -> (w31:dbl)
        n26 = local read "Q"() -> (w39:i32)
        n27 = local read "P"() -> (w40:i32)
        n28 = expression code="1+1e-6*p"(w28) -> (w27:dbl)
        n29 = To Double Precision Float(number=w40) -> (double precision float=w38:dbl)
        n30 = To Double Precision Float(number=w39) -> (double precision float=w37:dbl)
        n31 = expression code="1+p"(w33) -> (w32:dbl)
        n32 = Divide(x=w38, y=w37) -> (x/y=w36:dbl)
        n33 = Multiply(x=w31, y=w32) -> (x*y=w30:dbl)
        n34 = Compound Arithmetic op=MULTIPLY(w35, w36, w27) -> (w34:dbl)
        n35 = local write "max fs"(w30) -> ()
        n36 = local write "f0"(w34) -> ()
        n37 = local read "per mode"() -> (w29:bool)
        n38 = case shown="True" w29 {
          frame False {
            # "update period counts from integration times"
            n39 = local read "ref freq"() -> (w44:dbl)
            n40 = local read "max int"() -> (w46:dbl)
            n41 = local read "min int"() -> (w47:dbl)
            n42 = Build Array(w47, w46) -> (w45:dbl[])
            n43 = Multiply(x=w45, y=w44) -> (x*y=w43:dbl[])
            n44 = Index Array(array=w43) -> (element #1=w42:dbl, element #2=w41:dbl)  [unwired: 2 in]
            n45 = local write "min periods"(w42) -> ()
            n46 = local write "max periods"(w41) -> ()
          }
          frame True {
            # "update period counts from integration times"
            n47 = local read "max periods"() -> (w53:dbl)
            n48 = local read "min periods"() -> (w54:dbl)
            n49 = local read "ref freq"() -> (w51:dbl)
            n50 = Build Array(w54, w53) -> (w52:dbl[])
            n51 = Divide(x=w52, y=w51) -> (x/y=w50:dbl[])
            n52 = Index Array(array=w50) -> (element #1=w49:dbl, element #2=w48:dbl)  [unwired: 2 in]
            n53 = local write "min int"(w49) -> ()
            n54 = local write "max int"(w48) -> ()
          }
        }
      }
      event "btn ok", "btn cancel": Value Change; Panel Close {
        # "ok, cancel, exit"
        n55 = event-data() -> ()  [unwired: 1 in, 3 out]
        n56 = local read "smpl count"() -> (w70:i64)
        n57 = local read "found fs"() -> (w71:dbl)
        n58 = Bundle By Name(cluster=T1 {"fs [Hz]"=0.0, "N"=0, "error"=0.0} ("smpl setup"), "fs [Hz]"=w71, "N"=w70) -> (w69:T1)
        n59 = local write "smpl setup"(w69) -> ()
        n60 = local read "session out"() -> (w57:T2)
        n61 = local read "max fs rel tol"() -> (w63:dbl)
        n62 = local read "max timeout"() -> (w59:dbl)
        n63 = local read "ref freq"() -> (w65:dbl)
        n64 = local read "max err"() -> (w60:dbl)
        n65 = local read "rel shift"() -> (w66:dbl)
        n66 = local read "max int"() -> (w61:dbl)
        n67 = local read "min int"() -> (w62:dbl)
        n68 = local read "min fs"() -> (w64:dbl)
        n69 = local read "Q"() -> (w67:i32)
        n70 = local read "P"() -> (w68:i32)
        n71 = Unbundle By Name(w57) -> ("assist cfg"=w58:T67)
        n72 = Bundle By Name(cluster=w58, "P"=w68, "Q"=w67, "rel shift"=w66, "ref freq"=w65, "min fs"=w64, "max fs tol"=w63, "min int"=w62, "max int"=w61, "max err"=w60, "max timeout"=w59) -> (w56:T67)
        n73 = Bundle By Name(cluster=w57, "assist cfg"=w56) -> (w55:T2)
        n74 = local write "session out"(w55) -> ()
      }
      event "min int", "max int": Value Change {
        # "integration time update"
        n75 = event-data() -> ()  [unwired: 1 in, 6 out]
        n76 = local write "per mode"(FALSE ("per mode")) -> ()
      }
      event "min periods", "max periods": Value Change {
        # "periods count update"
        n77 = event-data() -> ()  [unwired: 1 in, 6 out]
        n78 = local write "per mode"(TRUE ("per mode")) -> ()
      }
      event "btn rough": Value Change {
        # "calculate rough sampling setup"
        n79 = event-data() -> ()  [unwired: 1 in, 6 out]
        n80 = local read "min periods"() -> (w87:dbl)
        n81 = local read "min fs"() -> (w84:dbl)
        n82 = local read "f0"() -> (w77:dbl)
        n83 = Divide(x=w87, y=w77) -> (x/y=w79:dbl)
        n84 = Multiply(x=w84, y=w79) -> (x*y=w86:dbl)
        n85 = To Long Integer(number=w86) -> (32bit integer=w83:i32)
        n86 = local write "found error"(nan ("found error")) -> ()
        n87 = local write "found fs"(w84) -> ()
        n88 = local write "found periods"(w87) -> ()
        n89 = local write "found int"(w79) -> ()
        n90 = local write "smpl count"(w83) -> ()
        n91 = To Double Precision Float(number=w83) -> (double precision float=w82:dbl)
        n92 = Divide(x=w84, y=w82) -> (x/y=w81:dbl)
        n93 = expression code="f*2"(w81) -> (w78:dbl)
        n94 = Divide(x=w77, y=w78) -> (x/y=w80:dbl)
        n95 = local write "found harm dist"(w80) -> ()
        n96 = local write "found bin step"(w78) -> ()
      }
      event "btn coh": Value Change {
        # "coherent setup finder"
        n97 = event-data() -> ()  [unwired: 1 in, 6 out]
        n98 = local read "session out"() -> (w106:T2)
        n99 = Unbundle By Name(w106) -> ("golpi"=w105:T55, "adc"=w104:T3)
        n100 = call "ADC Get Capabilities.vi"("adc session in"=w104) -> ("error out"=w103:errorcluster, "capabilities"=w102:T68)  [unwired: 8 in, 1 out]
        n101 = Unbundle By Name(w102) -> ("min fs [Hz]"=w101:ext, "max fs [Hz]"=w100:ext, "Ts step [s]"=w99:ext, "fs step [Hz]"=w98:ext, "smpl rate step mode"=w97:T69)
        n102 = local read "max fs rel tol"() -> (w90:dbl)
        n103 = local read "max timeout"() -> (w93:dbl)
        n104 = local read "max err"() -> (w92:dbl)
        n105 = local read "max int"() -> (w94:dbl)
        n106 = local read "min int"() -> (w95:dbl)
        n107 = local read "min fs"() -> (w91:dbl)
        n108 = local read "f0"() -> (w96:dbl)
        n109 = Bundle By Name(cluster=T70 {"fs min [Hz]"=0.0, "fs rel tol [-]"=0.0, "adc fs min [Hz]"=0.0, "adc fs max [Hz]"=0.0, "int min [s]"=0.0, "int max [s]"=0.0, "Ts step [s]"=0.0, "fs step [Hz]"=0.0, "timeout [s]"=0.0, "max err [-]"=0.0, "rate step mode"=enum."const period", "f0 [Hz]"=0.0} ("coherent finder setup"), "adc fs min [Hz]"=w101, "adc fs max [Hz]"=w100, "Ts step [s]"=w99, "fs step [Hz]"=w98, "rate step mode"=w97, "f0 [Hz]"=w96, "int min [s]"=w95, "int max [s]"=w94, "timeout [s]"=w93, "max err [-]"=w92, "fs min [Hz]"=w91, "fs rel tol [-]"=w90) -> (w107:T70)
        n110 = call "Assist Sampling Setup Calculate Coherent.vi"("golpi ref"=w105, "error in"=w103, "coherent finder setup"=w107) -> ("error out"=w89:errorcluster, "result"=w88:T1)  [unwired: 7 in]
        n111 = case shown="No Error" w89 {
          tunnel: w88 -> [w116 _]
          frame No Error {
            n112 = local write "smpl setup"(w116) -> ()
            n113 = Unbundle By Name(w116) -> ("error"=w115:dbl, "N"=w119:i64, "fs [Hz]"=w112:ext)
            n114 = local read "f0"() -> (w109:dbl)
            n115 = To Double Precision Float(number=w119) -> (double precision float=w111:dbl)
            n116 = Divide(x=w111, y=w112) -> (x/y=w118:ext)
            n117 = Divide(x=w112, y=w111) -> (x/y=w114:ext)
            n118 = expression code="f*2"(w114) -> (w110:ext)
            n119 = Multiply(x=w118, y=w109) -> (x*y=w117:ext)
            n120 = local write "smpl count"(w119) -> ()
            n121 = local write "found int"(w118) -> ()
            n122 = local write "found fs"(w112) -> ()
            n123 = local write "found error"(w115) -> ()
            n124 = local write "found periods"(w117) -> ()
            n125 = Divide(x=w109, y=w110) -> (x/y=w113:ext)
            n126 = local write "found bin step"(w110) -> ()
            n127 = local write "found harm dist"(w113) -> ()
          }
          frame Error {
          }
        }
      }
      event "btn meas": Value Change {
        # "MEASURE REFERENCE FREQ"
        n128 = event-data() -> ()  [unwired: 1 in, 6 out]
        n129 = call "Assist Sampling Measure Freq Panel.vi"() -> ("error out"=w122:errorcluster, "confirmed?"=w121:bool, "meas f avg"=w120:dbl)  [unwired: 9 in]
        n130 = case shown="True" w121 {
          tunnel: w120 -> [_ w123]
          frame False {
          }
          frame True {
            n131 = local write "ref freq"(w123) -> ()
          }
        }
        n132 = local write "error out"(w122) -> ()
      }
    }
  }
  "ok" <- w17
  "session out" <- "session in"
  "per mode" <- FALSE ("per mode")
